vi "Update Album.vi"(7 "Album ID":T1 caption="인덱스 값", 8 "error in (no error)":errorcluster, 9 "Artist ID":i64, 10 "Name":string, 11 "SQLite Connection in":refnum<class "Connection.lvclass">) -> (0 "error out":errorcluster, 3 "SQLite Connection out":refnum<class "Connection.lvclass">)   [LabVIEW 2015]
uses:
  <vilib>/drjdpowell/SQLite Library/SQL Connection/Connection.lvclass
  <vilib>/Utility/miscctls.llb/LVRowAndColumnUnsignedTypeDef.ctl
  <vilib>/drjdpowell/SQLite Library/SQL Statement/SQL Statement.lvclass/SQL Statement.ctl
  <vilib>/drjdpowell/SQLite Library/SQL Statement/Bind Text.vi
  <vilib>/drjdpowell/SQLite Library/SQL Statement/Bind Integer.vi
  <vilib>/drjdpowell/SQLite Library/SQL Statement/Step.vi
  <vilib>/drjdpowell/SQLite Library/SQL Statement/Error Message.vi
  <vilib>/drjdpowell/SQLite Library/SQL Statement/SQL Statement.lvclass
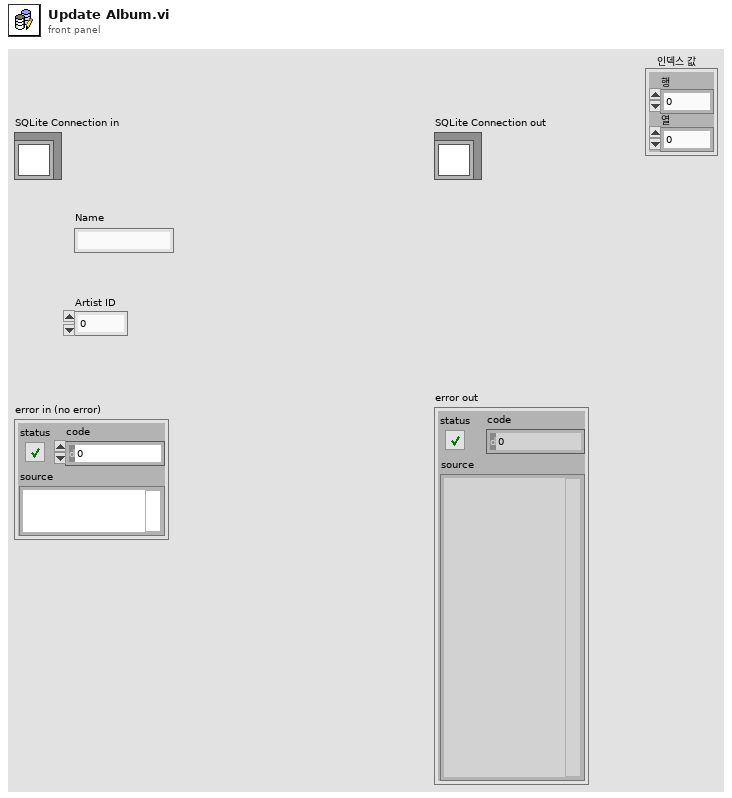
[diagram p1: front panel]
types:
  T1 = typedef "LVRowAndColumnUnsignedTypeDef.ctl" = cluster{"Row":u32, "Column":u32}
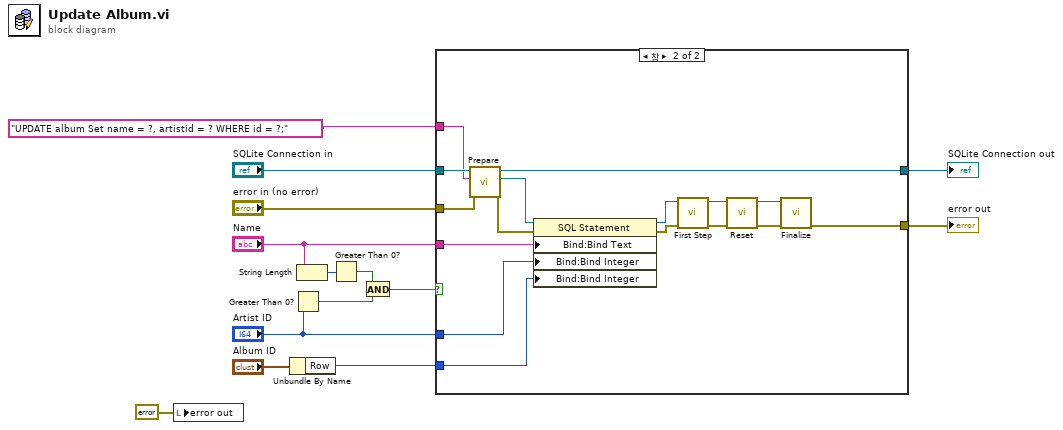
[diagram p0: block diagram]
diagram:
  n1 = local write "error out"(errorcluster {"status"=FALSE, "code"=0, "source"=""} ("error in (no error) 2")) -> ()
  n2 = Unbundle By Name("Album ID") -> ("Row"=w2:u32)
  n3 = Greater Than 0?(x="Artist ID") -> (x > 0?=w12:bool)
  n4 = String Length(string="Name") -> (length=w14:i32)
  n5 = Greater Than 0?(x=w14) -> (x > 0?=w13:bool)
  n6 = And(x=w13, y=w12) -> (x .and. y?=w11:bool)
  n7 = case shown="참" w11 {
    tunnel: "SQLite Connection in" -> [w16 w32]
    tunnel: "error in (no error)" -> [w15 w31]
    tunnel: "UPDATE album Set name = ?, artistid = ? WHERE id = ?;" -> [_ w30]
    tunnel: "Name" -> [_ w27]
    tunnel: "Artist ID" -> [_ w26]
    tunnel: [w16 w19] -> w5
    tunnel: [w15 w18] -> w4
    tunnel: w2 -> [_ w17]
    frame False {
    }
    frame True {
      n8 = call <vilib>:"Prepare.vi"("error in (no error)"=w31, "SQL"=w30, "SQLite Connection in"=w32) -> ("error out"=w29:errorcluster, "SQL Statement"=w28:refnum<class "SQL Statement.lvclass">, "SQLite Connection"=w19:refnum<class "Connection.lvclass">)  [unwired: 4 in, 2 out]
      n9 = property class="SQL Statement"(reference=w28, error in=w29, "Bind:Bind Text"=w27, "Bind:Bind Integer"=w26, "Bind:Bind Integer"=w17) -> (reference out=w24:refnum<class "SQL Statement.lvclass">, error out=w25:errorcluster)
      n10 = call <vilib>:"First Step.vi"("error in (no error)"=w25, "SQL Statement in"=w24) -> ("error out"=w22:errorcluster, "SQL Statement"=w23:refnum<class "SQL Statement.lvclass">)  [unwired: 7 in, 1 out]
      n11 = call <vilib>:"Reset.vi"("error in (no error)"=w22, "SQL Statement in"=w23) -> ("error out"=w21:errorcluster, "SQL Statement"=w20:refnum<class "SQL Statement.lvclass">)  [unwired: 8 in]
      n12 = call <vilib>:"Finalize.vi"("error in (no error)"=w21, "SQL Statement in"=w20) -> ("error out"=w18:errorcluster)  [unwired: 9 in]
    }
  }
  "SQLite Connection out" <- w5
  "error out" <- w4
